vi "Check and Create Dir for data save.vi"(0 "Path In":path=path "F:/1/2/4.txt", 11 "Error In":errorcluster) -> (4 "Dup Path Out":path=path "F:/1", 6 "Insert Name 2":bool, 15 "Error Out":errorcluster)   [LabVIEW 2015]
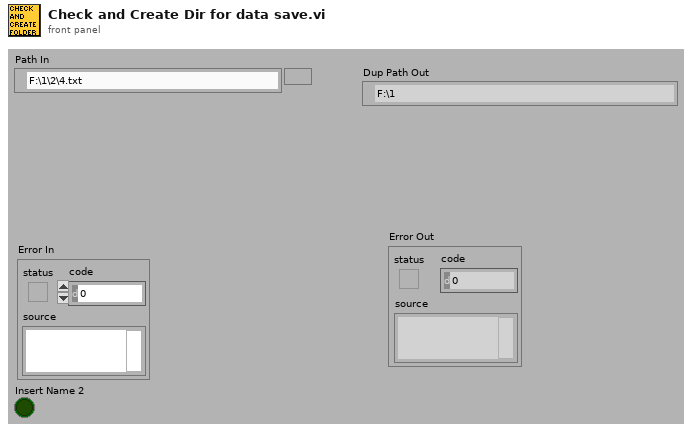
[diagram p1: front panel]
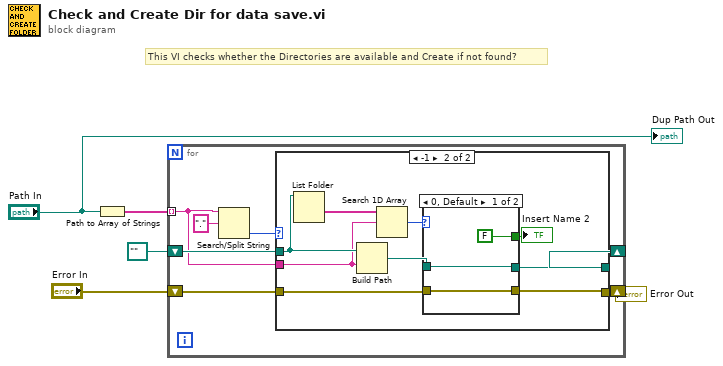
[diagram p0: block diagram]
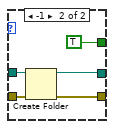
[diagram p3: hidden frame]
diagram:
  # "This VI checks whether the Directories are available and Create if not found?"
  n1 = Path to Array of Strings(0:"Path In") -> (2:w4:string[])  [unwired: 1 out]
  n2 = for {
    tunnel: w4 -> [w9] mode=indexing
    shift-right: [w8] -> _
    shift-left: path "" ("Path Out") -> [w10]
    shift-right: [w6] -> w1
    shift-left: "Error In" -> [w7]
    n3 = Search/Split String(string=w9, search string/char (-)=".") -> (offset of match=w11:i32)  [unwired: 3 out]
    n4 = case shown="-1" w11 {
      tunnel: w10 -> [w14 w21]
      tunnel: w9 -> [_ w18]
      tunnel: [w14 w23] -> w8
      tunnel: w7 -> [w13 w17]
      tunnel: [w13 w16] -> w6
      frame 0, Default {
      }
      frame -1 {
        n5 = List Folder(path=w21) -> (folder names=w19:string[])  [unwired: 1 in, 5 out]
        n6 = Build Path(base path=w21, name or relative path=w18) -> (appended path=w22:path)
        n7 = Search 1D Array(1D array=w19, element=w18) -> (index of element=w20:i32)  [unwired: 1 out]
        n8 = case shown="0, Default" w20 {
          tunnel: [w26 w31] -> w23
          tunnel: w22 -> [w26 w30]
          tunnel: w17 -> [w25 w29]
          tunnel: [w25 w28] -> w16
          tunnel: [FALSE TRUE] -> w15
          frame 0, Default {
          }
          frame -1 {
            n9 = Create Folder(path (use dialog)=w30, error in=w29) -> (created path=w31:path, error out=w28:errorcluster)  [unwired: 2 out]
          }
        }
        "Insert Name 2" <- w15
      }
    }
  }
  "Error Out" <- w1
  "Dup Path Out" <- "Path In"
